vi "Wizard 2D Array sort - String.vi"(2 "error in (no error)":errorcluster, 3 "Array In":string[][](array[string])) -> (0 "error out":errorcluster, 1 "Array Out":string[][](array[string]))   [LabVIEW 2014]
doc: "<B>Copyright</B>: (c) 2015 MHWirth. Modified version of original developed by (Toby Stensland, toby@labjack.com, LabJack Corporation, www.labjack.com)\n\nThis subVI alphabetically sorts a 2D array of strings based on the first column. \n\n<B>Limitation</B> Number of columns is limited to 255."
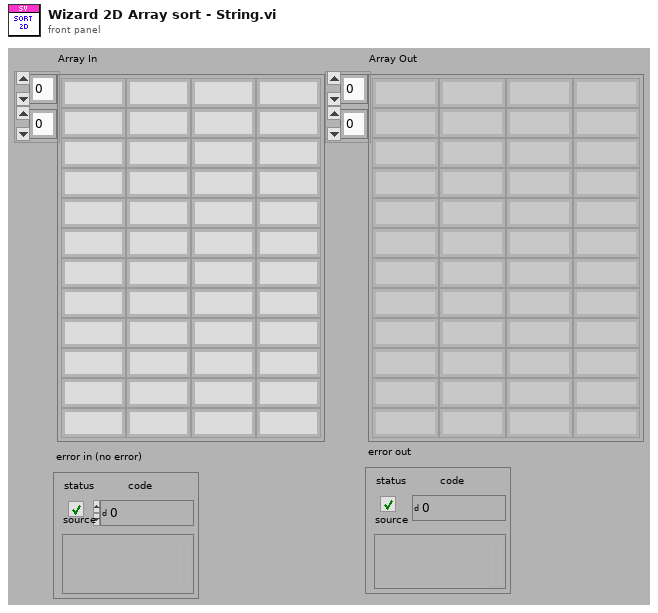
[diagram p1: front panel]
types:
  T1 = cluster{"Array In[0]":string, "Array In[1]":string, "Array In[2]":string, "Array In[3]":string, "Array In[4]":string, "Array In[5]":string, "Array In[6]":string, "Array In[7]":string, "Array In[8]":string, "Array In[9]":string, "Array In[10]":string, "Array In[11]":string, "Array In[12]":string, "Array In[13]":string, "Array In[14]":string, "Array In[15]":string, "Array In[16]":string, "Array In[17]":string, "Array In[18]":string, "Array In[19]":string, "Array In[20]":string, "Array In[21]":string, "Array In[22]":string, "Array In[23]":string, "Array In[24]":string, "Array In[25]":string, "Array In[26]":string, "Array In[27]":string, "Array In[28]":string, "Array In[29]":string, "Array In[30]":string, "Array In[31]":string, "Array In[32]":string, "Array In[33]":string, "Array In[34]":string, "Array In[35]":string, "Array In[36]":string, "Array In[37]":string, "Array In[38]":string, "Array In[39]":string, "Array In[40]":string, "Array In[41]":string, "Array In[42]":string, "Array In[43]":string, "Array In[44]":string, "Array In[45]":string, "Array In[46]":string, "Array In[47]":string, "Array In[48]":string, "Array In[49]":string, "Array In[50]":string, "Array In[51]":string, "Array In[52]":string, "Array In[53]":string, "Array In[54]":string, "Array In[55]":string, "Array In[56]":string, "Array In[57]":string, "Array In[58]":string, "Array In[59]":string, "Array In[60]":string, "Array In[61]":string, "Array In[62]":string, "Array In[63]":string, "Array In[64]":string, "Array In[65]":string, "Array In[66]":string, "Array In[67]":string, "Array In[68]":string, "Array In[69]":string, "Array In[70]":string, "Array In[71]":string, "Array In[72]":string, "Array In[73]":string, "Array In[74]":string, "Array In[75]":string, "Array In[76]":string, "Array In[77]":string, "Array In[78]":string, "Array In[79]":string, "Array In[80]":string, "Array In[81]":string, "Array In[82]":string, "Array In[83]":string, "Array In[84]":string, "Array In[85]":string, "Array In[86]":string, "Array In[87]":string, "Array In[88]":string, "Array In[89]":string, "Array In[90]":string, "Array In[91]":string, "Array In[92]":string, "Array In[93]":string, "Array In[94]":string, "Array In[95]":string, "Array In[96]":string, "Array In[97]":string, "Array In[98]":string, "Array In[99]":string, "Array In[100]":string, "Array In[101]":string, "Array In[102]":string, "Array In[103]":string, "Array In[104]":string, "Array In[105]":string, "Array In[106]":string, "Array In[107]":string, "Array In[108]":string, "Array In[109]":string, "Array In[110]":string, "Array In[111]":string, "Array In[112]":string, "Array In[113]":string, "Array In[114]":string, "Array In[115]":string, "Array In[116]":string, "Array In[117]":string, "Array In[118]":string, "Array In[119]":string, "Array In[120]":string, "Array In[121]":string, "Array In[122]":string, "Array In[123]":string, "Array In[124]":string, "Array In[125]":string, "Array In[126]":string, "Array In[127]":string, "Array In[128]":string, "Array In[129]":string, "Array In[130]":string, "Array In[131]":string, "Array In[132]":string, "Array In[133]":string, "Array In[134]":string, "Array In[135]":string, "Array In[136]":string, "Array In[137]":string, "Array In[138]":string, "Array In[139]":string, "Array In[140]":string, "Array In[141]":string, "Array In[142]":string, "Array In[143]":string, "Array In[144]":string, "Array In[145]":string, "Array In[146]":string, "Array In[147]":string, "Array In[148]":string, "Array In[149]":string, "Array In[150]":string, "Array In[151]":string, "Array In[152]":string, "Array In[153]":string, "Array In[154]":string, "Array In[155]":string, "Array In[156]":string, "Array In[157]":string, "Array In[158]":string, "Array In[159]":string, "Array In[160]":string, "Array In[161]":string, "Array In[162]":string, "Array In[163]":string, "Array In[164]":string, "Array In[165]":string, "Array In[166]":string, "Array In[167]":string, "Array In[168]":string, "Array In[169]":string, "Array In[170]":string, "Array In[171]":string, "Array In[172]":string, "Array In[173]":string, "Array In[174]":string, "Array In[175]":string, "Array In[176]":string, "Array In[177]":string, "Array In[178]":string, "Array In[179]":string, "Array In[180]":string, "Array In[181]":string, "Array In[182]":string, "Array In[183]":string, "Array In[184]":string, "Array In[185]":string, "Array In[186]":string, "Array In[187]":string, "Array In[188]":string, "Array In[189]":string, "Array In[190]":string, "Array In[191]":string, "Array In[192]":string, "Array In[193]":string, "Array In[194]":string, "Array In[195]":string, "Array In[196]":string, "Array In[197]":string, "Array In[198]":string, "Array In[199]":string, "Array In[200]":string, "Array In[201]":string, "Array In[202]":string, "Array In[203]":string, "Array In[204]":string, "Array In[205]":string, "Array In[206]":string, "Array In[207]":string, "Array In[208]":string, "Array In[209]":string, "Array In[210]":string, "Array In[211]":string, "Array In[212]":string, "Array In[213]":string, "Array In[214]":string, "Array In[215]":string, "Array In[216]":string, "Array In[217]":string, "Array In[218]":string, "Array In[219]":string, "Array In[220]":string, "Array In[221]":string, "Array In[222]":string, "Array In[223]":string, "Array In[224]":string, "Array In[225]":string, "Array In[226]":string, "Array In[227]":string, "Array In[228]":string, "Array In[229]":string, "Array In[230]":string, "Array In[231]":string, "Array In[232]":string, "Array In[233]":string, "Array In[234]":string, "Array In[235]":string, "Array In[236]":string, "Array In[237]":string, "Array In[238]":string, "Array In[239]":string, "Array In[240]":string, "Array In[241]":string, "Array In[242]":string, "Array In[243]":string, "Array In[244]":string, "Array In[245]":string, "Array In[246]":string, "Array In[247]":string, "Array In[248]":string, "Array In[249]":string, "Array In[250]":string, "Array In[251]":string, "Array In[252]":string, "Array In[253]":string, "Array In[254]":string, "Array In[255]":string}
  T2 = cluster{"Array In[0]":string, "Array In[1]":string, "Array In[2]":string, "Array In[3]":string, "Array In[4]":string, "Array In[5]":string, "Array In[6]":string, "Array In[7]":string, "Array In[8]":string, "Array In[9]":string, "Array In[10]":string, "Array In[11]":string, "Array In[12]":string, "Array In[13]":string, "Array In[14]":string, "Array In[15]":string, "Array In[16]":string, "Array In[17]":string, "Array In[18]":string, "Array In[19]":string, "Array In[20]":string, "Array In[21]":string, "Array In[22]":string, "Array In[23]":string, "Array In[24]":string, "Array In[25]":string, "Array In[26]":string, "Array In[27]":string, "Array In[28]":string, "Array In[29]":string, "Array In[30]":string, "Array In[31]":string, "Array In[32]":string, "Array In[33]":string, "Array In[34]":string, "Array In[35]":string, "Array In[36]":string, "Array In[37]":string, "Array In[38]":string, "Array In[39]":string, "Array In[40]":string, "Array In[41]":string, "Array In[42]":string, "Array In[43]":string, "Array In[44]":string, "Array In[45]":string, "Array In[46]":string, "Array In[47]":string, "Array In[48]":string, "Array In[49]":string, "Array In[50]":string, "Array In[51]":string, "Array In[52]":string, "Array In[53]":string, "Array In[54]":string, "Array In[55]":string, "Array In[56]":string, "Array In[57]":string, "Array In[58]":string, "Array In[59]":string, "Array In[60]":string, "Array In[61]":string, "Array In[62]":string, "Array In[63]":string, "Array In[64]":string, "Array In[65]":string, "Array In[66]":string, "Array In[67]":string, "Array In[68]":string, "Array In[69]":string, "Array In[70]":string, "Array In[71]":string, "Array In[72]":string, "Array In[73]":string, "Array In[74]":string, "Array In[75]":string, "Array In[76]":string, "Array In[77]":string, "Array In[78]":string, "Array In[79]":string, "Array In[80]":string, "Array In[81]":string, "Array In[82]":string, "Array In[83]":string, "Array In[84]":string, "Array In[85]":string, "Array In[86]":string, "Array In[87]":string, "Array In[88]":string, "Array In[89]":string, "Array In[90]":string, "Array In[91]":string, "Array In[92]":string, "Array In[93]":string, "Array In[94]":string, "Array In[95]":string, "Array In[96]":string, "Array In[97]":string, "Array In[98]":string, "Array In[99]":string, "Array In[100]":string, "Array In[101]":string, "Array In[102]":string, "Array In[103]":string, "Array In[104]":string, "Array In[105]":string, "Array In[106]":string, "Array In[107]":string, "Array In[108]":string, "Array In[109]":string, "Array In[110]":string, "Array In[111]":string, "Array In[112]":string, "Array In[113]":string, "Array In[114]":string, "Array In[115]":string, "Array In[116]":string, "Array In[117]":string, "Array In[118]":string, "Array In[119]":string, "Array In[120]":string, "Array In[121]":string, "Array In[122]":string, "Array In[123]":string, "Array In[124]":string, "Array In[125]":string, "Array In[126]":string, "Array In[127]":string, "Array In[128]":string, "Array In[129]":string, "Array In[130]":string, "Array In[131]":string, "Array In[132]":string, "Array In[133]":string, "Array In[134]":string, "Array In[135]":string, "Array In[136]":string, "Array In[137]":string, "Array In[138]":string, "Array In[139]":string, "Array In[140]":string, "Array In[141]":string, "Array In[142]":string, "Array In[143]":string, "Array In[144]":string, "Array In[145]":string, "Array In[146]":string, "Array In[147]":string, "Array In[148]":string, "Array In[149]":string, "Array In[150]":string, "Array In[151]":string, "Array In[152]":string, "Array In[153]":string, "Array In[154]":string, "Array In[155]":string, "Array In[156]":string, "Array In[157]":string, "Array In[158]":string, "Array In[159]":string, "Array In[160]":string, "Array In[161]":string, "Array In[162]":string, "Array In[163]":string, "Array In[164]":string, "Array In[165]":string, "Array In[166]":string, "Array In[167]":string, "Array In[168]":string, "Array In[169]":string, "Array In[170]":string, "Array In[171]":string, "Array In[172]":string, "Array In[173]":string, "Array In[174]":string, "Array In[175]":string, "Array In[176]":string, "Array In[177]":string, "Array In[178]":string, "Array In[179]":string, "Array In[180]":string, "Array In[181]":string, "Array In[182]":string, "Array In[183]":string, "Array In[184]":string, "Array In[185]":string, "Array In[186]":string, "Array In[187]":string, "Array In[188]":string, "Array In[189]":string, "Array In[190]":string, "Array In[191]":string, "Array In[192]":string, "Array In[193]":string, "Array In[194]":string, "Array In[195]":string, "Array In[196]":string, "Array In[197]":string, "Array In[198]":string, "Array In[199]":string, "Array In[200]":string, "Array In[201]":string, "Array In[202]":string, "Array In[203]":string, "Array In[204]":string, "Array In[205]":string, "Array In[206]":string, "Array In[207]":string, "Array In[208]":string, "Array In[209]":string, "Array In[210]":string, "Array In[211]":string, "Array In[212]":string, "Array In[213]":string, "Array In[214]":string, "Array In[215]":string, "Array In[216]":string, "Array In[217]":string, "Array In[218]":string, "Array In[219]":string, "Array In[220]":string, "Array In[221]":string, "Array In[222]":string, "Array In[223]":string, "Array In[224]":string, "Array In[225]":string, "Array In[226]":string, "Array In[227]":string, "Array In[228]":string, "Array In[229]":string, "Array In[230]":string, "Array In[231]":string, "Array In[232]":string, "Array In[233]":string, "Array In[234]":string, "Array In[235]":string, "Array In[236]":string, "Array In[237]":string, "Array In[238]":string, "Array In[239]":string, "Array In[240]":string, "Array In[241]":string, "Array In[242]":string, "Array In[243]":string, "Array In[244]":string, "Array In[245]":string, "Array In[246]":string, "Array In[247]":string, "Array In[248]":string, "Array In[249]":string, "Array In[250]":string, "Array In[251]":string, "Array In[252]":string, "Array In[253]":string, "Array In[254]":string, "Array In[255]":string}[]
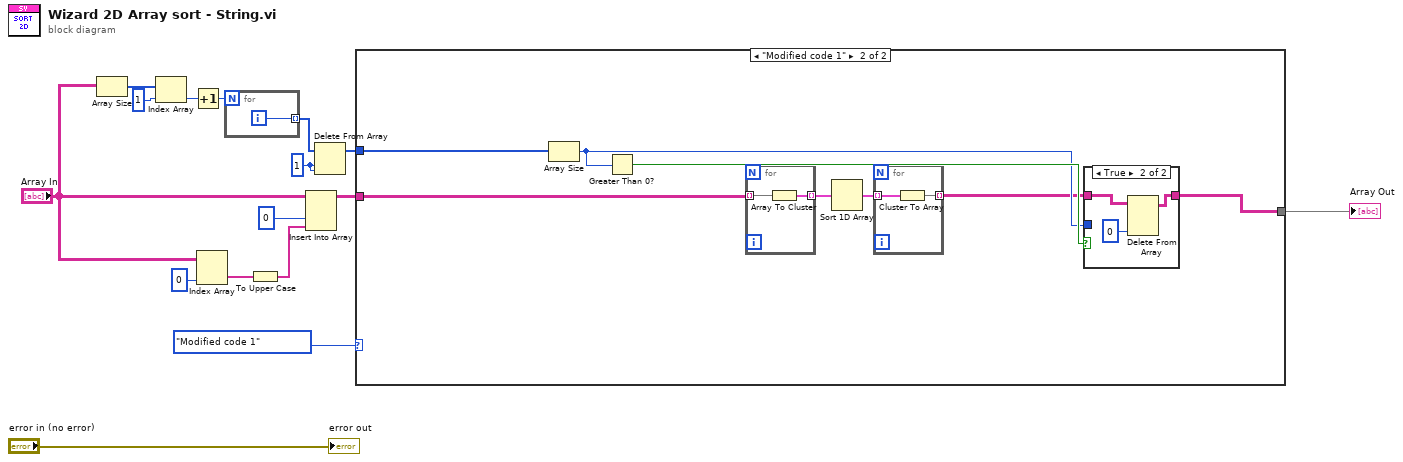
[diagram p0: block diagram]
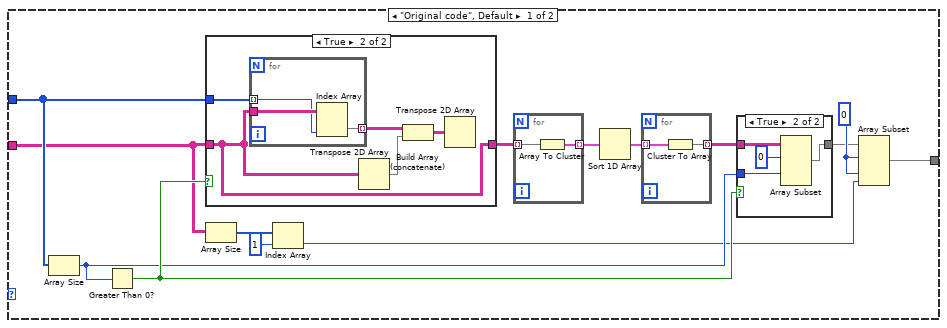
[diagram p2: hidden frame]
diagram:
  w14 = 1 ("Index")
  n1 = Array Size(array="Array In") -> (size(s)=w11:i32[])
  n2 = Index Array(array=w11, index=1 ("Array Index")) -> (element=w13:i32)
  n3 = Increment(x=w13) -> (x+1=w10:i32)
  n4 = Index Array(array="Array In", index (col)=0 ("disabled index (col)")) -> (element=w7:string[])  [unwired: 1 in]
  n5 = for {
    N: w10 -> [_]
    tunnel: [w17] -> w9 mode=indexing
    i -> [w17]
  }
  n6 = To Upper Case(1:w7) -> (0:w6:string[])
  n7 = Insert Into Array(array="Array In", index (col)=0 ("disabled index (col)"), new element=w6) -> (w5:string[][])  [unwired: 1 in]
  n8 = Delete From Array(array=w9, length=w14, index=w14) -> (array with subset deleted=w8:i32[])  [unwired: 1 out]
  n9 = case shown="\"Modified code 1\"" enum16{"Original code", "Modified code 1"}."Modified code 1" {
    tunnel: w8 -> [w31 w57]
    tunnel: w5 -> [w29 w50]
    tunnel: [w24 w51] -> w16
    frame "Original code", Default {
      w20 = 0 ("Array Index")
      n10 = Array Size(array=w31) -> (size(s)=w26:i32)
      n11 = Greater Than 0?(x=w26) -> (x > 0?=w30:bool)
      n12 = case shown="True" w30 {
        tunnel: w31 -> [_ w42]
        tunnel: w29 -> [w37 w38]
        tunnel: [w37 w38] -> w21
        frame False {
        }
        frame True {
          n13 = for {
            tunnel: w42 -> [w44] mode=indexing
            tunnel: w38 -> [w45]
            tunnel: [w43] -> w41 mode=indexing
            n14 = Index Array(array=w45, index (col)=w44) -> (element=w43:string[])  [unwired: 1 in]
          }
          n15 = Transpose 2D Array(2D array=w38) -> (transposed array=w40:string[][])
          n16 = Build Array (concatenate)(w41, w40) -> (w39:string[][])
          n17 = Transpose 2D Array(2D array=w39) -> ()  [unwired: 1 out]
        }
      }
      n18 = Array Size(array=w29) -> (size(s)=w28:i32[])
      n19 = Index Array(array=w28, index=1 ("Index")) -> (element=w25:i32)
      n20 = for {
        tunnel: w21 -> [w49] mode=indexing
        tunnel: [w48] -> w23 mode=indexing
        n21 = Array To Cluster(array=w49) -> (cluster=w48:T1)
      }
      n22 = Sort 1D Array(array=w23) -> (sorted array=w22:T2)
      n23 = for {
        tunnel: w22 -> [w47] mode=indexing
        tunnel: [w46] -> w19 mode=indexing
        n24 = Cluster To Array(cluster=w47) -> (array=w46:string[])
      }
      n25 = case shown="True" w30 {
        tunnel: [w32 w33] -> w18
        tunnel: w19 -> [w32 w36]
        tunnel: w26 -> [_ w35]
        frame False {
        }
        frame True {
          n26 = Array Subset(array=w36, index (row)=0 ("Array Index"), index (col)=w35) -> (w33:string[][])  [unwired: 2 in]
        }
      }
      n27 = Array Subset(array=w18, index (row)=w20, index (col)=w20, length (col)=w25) -> (w24:string[][])  [unwired: 1 in]
    }
    frame "Modified code 1" {
      n28 = Array Size(array=w57) -> (size(s)=w55:i32)
      n29 = Greater Than 0?(x=w55) -> (x > 0?=w56:bool)
      n30 = for {
        tunnel: w50 -> [w65] mode=indexing
        tunnel: [w64] -> w54 mode=indexing
        n31 = Array To Cluster(array=w65) -> (cluster=w64:T1)
      }
      n32 = Sort 1D Array(array=w54) -> (sorted array=w53:T2)
      n33 = for {
        tunnel: w53 -> [w63] mode=indexing
        tunnel: [w62] -> w52 mode=indexing
        n34 = Cluster To Array(cluster=w63) -> (array=w62:string[])
      }
      n35 = case shown="True" w56 {
        tunnel: [w58 w59] -> w51
        tunnel: w52 -> [w58 w61]
        tunnel: w55 -> [_ _]
        frame False {
        }
        frame True {
          n36 = Delete From Array(array=w61, index (col)=0 ("disabled index (col)")) -> (array with subset deleted=w59:string[][])  [unwired: 2 in, 1 out]
        }
      }
    }
  }
  "Array Out" <- w16
  "error out" <- "error in (no error)"
